vi "Modbus Master example merged.vi"() -> ()   [LabVIEW 2020, in "Modbus.lvlib"]
uses:
  Modbus.lvlib
  <vilib>/NI/Modbus Library/API/Master/Modbus Master.lvclass
  <vilib>/NI/Modbus Library/Master Function Definition/Read Device ID code.ctl
  <vilib>/NI/Modbus Library/API/Wrapper/Create TCP Master.vi
  <vilib>/NI/Modbus Library/API/Wrapper/API Main.lvlib
  <vilib>/NI/Modbus Library/Data Model/Device Data Model.lvclass
panel:
  out "Command PLC to spill gasoline can":bool
  out "Connected state":bool
  in  "Command PLC to spil gasoline can":bool
  in  "Holding Registers":u16[](array[numeric])=[0, 0, 0, 0, 0, 0, 0, 0]
  in  "Coils":bool[](array[boolean])=[FALSE, FALSE, FALSE, FALSE, FALSE, FALSE, FALSE, FALSE]
  out "Discrete Inputs":bool[](array[boolean])
  out "Input Registers":u16[](array[numeric])
  out "Basic Objects":string[](array[string])
  in  "Slave Address":string="localhost"
  in  "Port":u16=502
  out "Status":string
  in  "Stop Button":bool
  in  "Set Holding Registers":bool
  in  "Set Coils":bool
  in  "Fetch Discrete Inputs":bool
  in  "Fetch Input Registers":bool
  in  "Fetch Basic Objects":bool
  in  "Disconnect":bool
  in  "Connect":bool
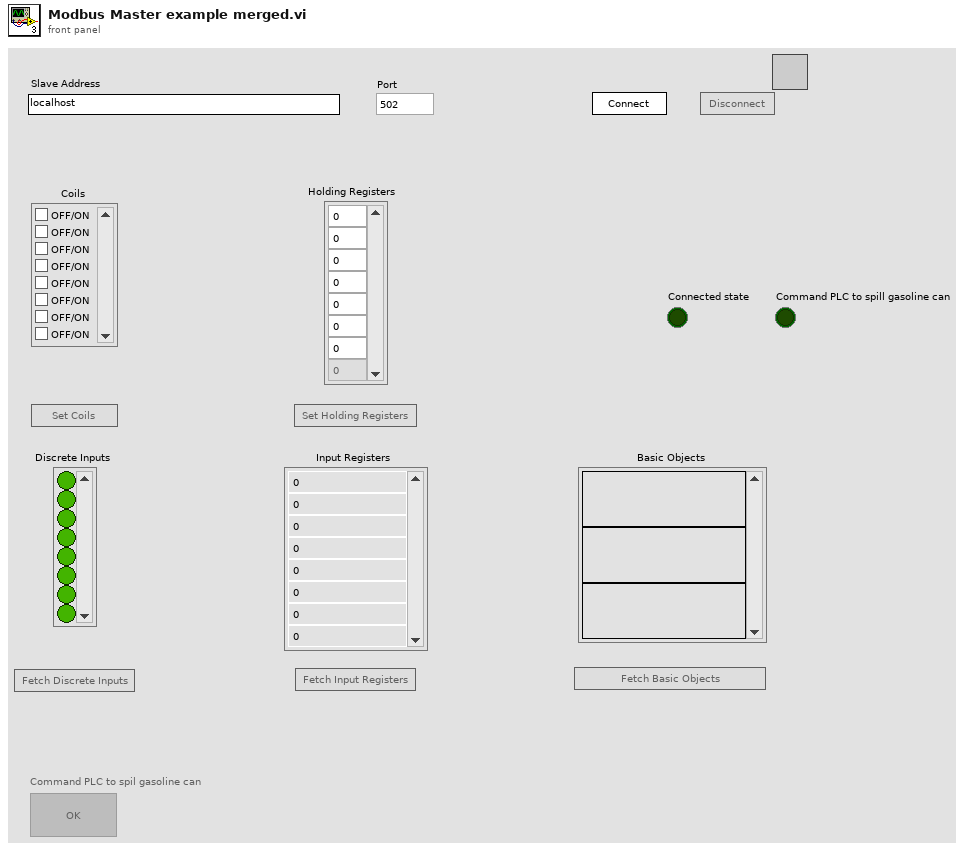
[diagram p1: front panel]
types:
  T1 = enum8{"Enabled", "Disabled", "Disabled and Grayed Out"}
  T2 = typedef "Device Data Model.lvclass/Read Device ID code.ctl" = enum8{"Read Basic", "Read Regular", "Read Extended", "Read Specific"}
  T3 = typedef "Device Data Model.lvclass/Identification Parameters.ctl" = cluster{"Object ID":u8, "Value":string}
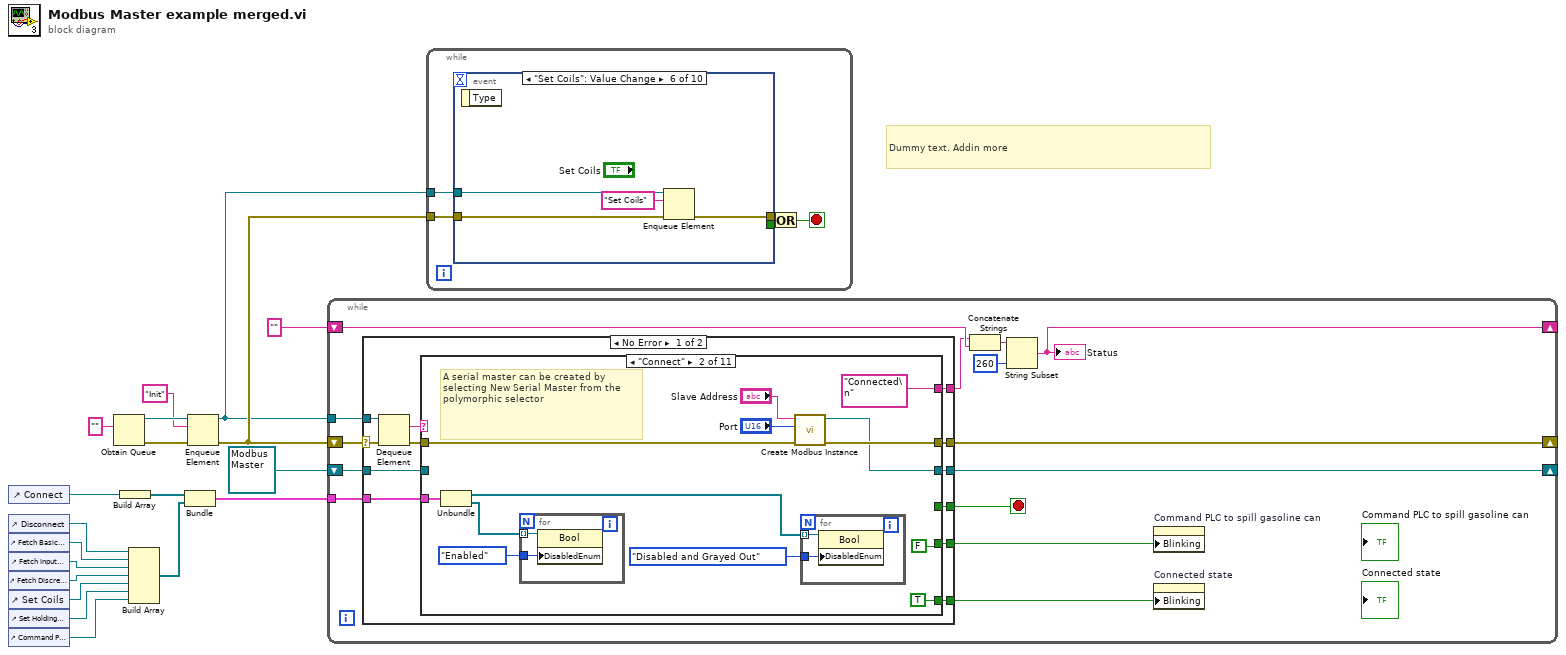
[diagram p0: block diagram]
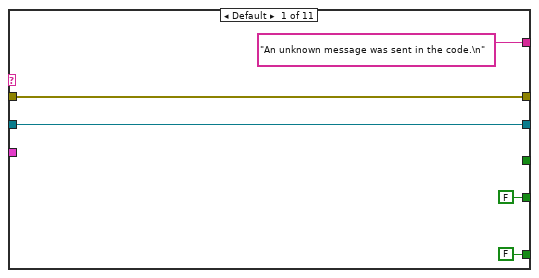
[diagram p2: hidden frame]
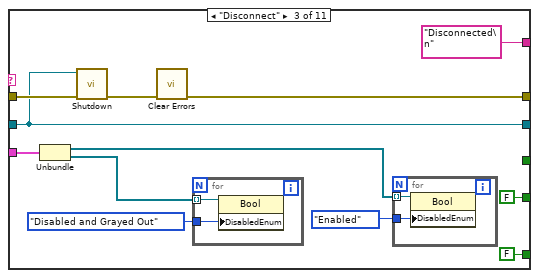
[diagram p3: hidden frame]
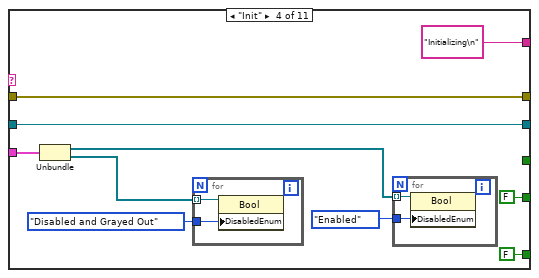
[diagram p4: hidden frame]
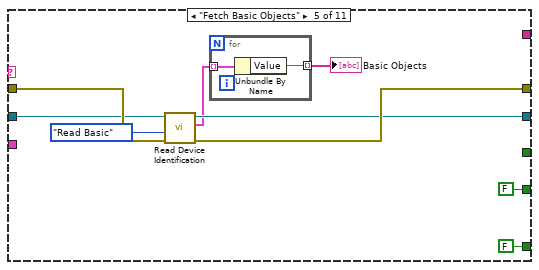
[diagram p5: hidden frame]
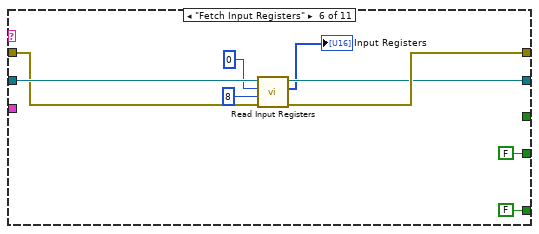
[diagram p6: hidden frame]
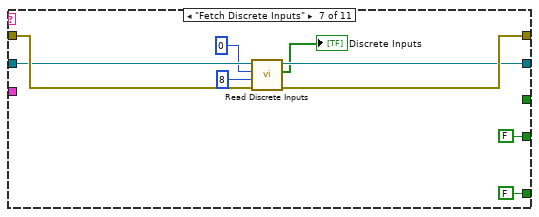
[diagram p7: hidden frame]
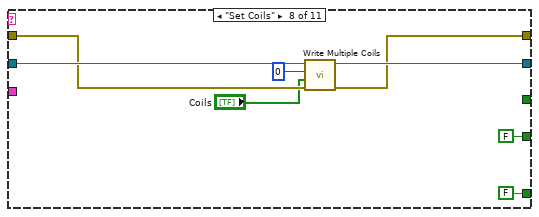
[diagram p8: hidden frame]
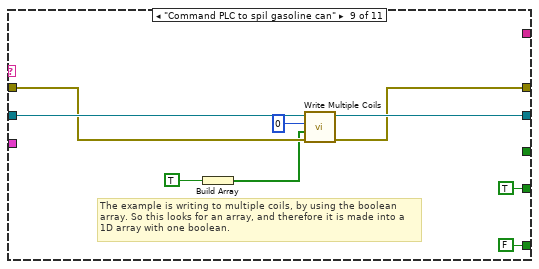
[diagram p9: hidden frame]
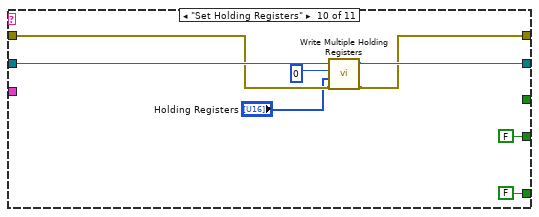
[diagram p10: hidden frame]
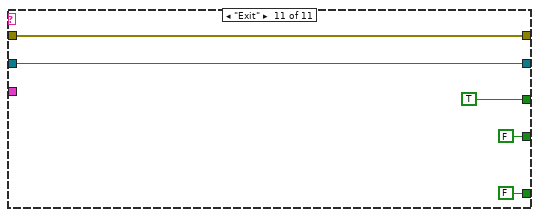
[diagram p11: hidden frame]
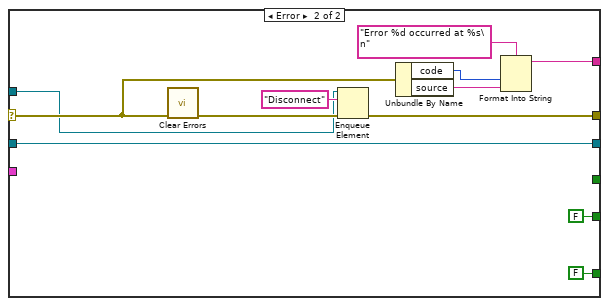
[diagram p12: hidden frame]
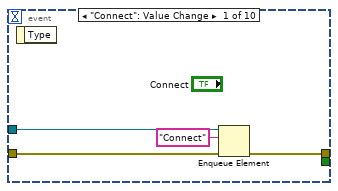
[diagram p13: hidden frame]
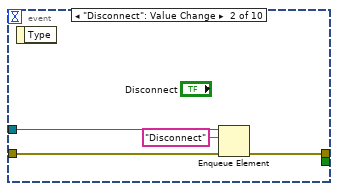
[diagram p14: hidden frame]
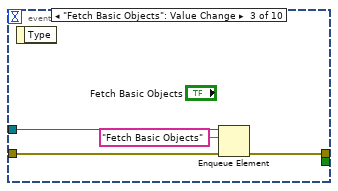
[diagram p15: hidden frame]
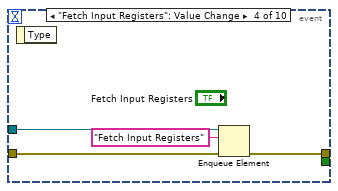
[diagram p16: hidden frame]
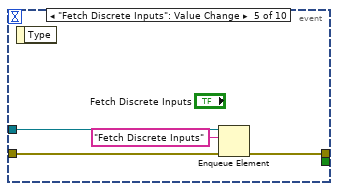
[diagram p17: hidden frame]
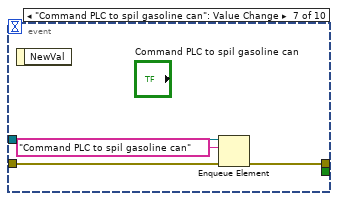
[diagram p18: hidden frame]
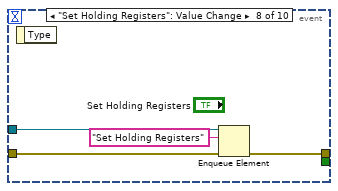
[diagram p19: hidden frame]
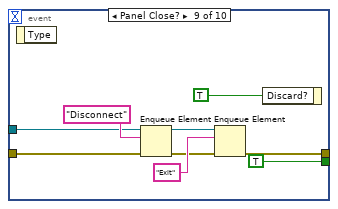
[diagram p20: hidden frame]
diagram:
  # "Dummy text. Addin more"
  n1 = control-ref of="Connect"() -> (w10:refnum<vi>)
  n2 = control-ref of="Disconnect"() -> (w16:refnum<vi>)
  n3 = control-ref of="Fetch Basic Objects"() -> (w15:refnum<vi>)
  n4 = control-ref of="Fetch Input Registers"() -> (w14:refnum<vi>)
  n5 = control-ref of="Fetch Discrete Inputs"() -> (w13:refnum<vi>)
  n6 = control-ref of="Set Coils"() -> (w12:refnum<vi>)
  n7 = control-ref of="Set Holding Registers"() -> (w11:refnum<vi>)
  n8 = control-ref of="Command PLC to spil gasoline can"() -> (w1:refnum<vi>)
  n9 = Obtain Queue(element data type="") -> (queue out=w5:refnum<queue>, error out=w19:errorcluster)  [unwired: 4 in, 1 out]
  n10 = Build Array(w10) -> (w7:refnum<vi>[])
  n11 = Build Array(w16, w15, w14, w13, w12, w11, w1) -> (w9:refnum<vi>[])
  n12 = Bundle(w7, w9) -> (w8:cluster{refnum<vi>[], refnum<vi>[]})  [unwired: 1 in]
  n13 = Enqueue Element(queue=w5, element="Init", error in (no error)=w19) -> (queue out=w4:refnum<queue>, error out=w6:errorcluster)  [unwired: 1 in, 1 out]
  n14 = while {
    shift-right: [w25] -> _
    shift-left: refnum<class "Modbus Master.lvclass"> refnum ("Modbus Master") -> [w24]
    tunnel: w4 -> [w33]
    shift-right: [w31] -> _
    shift-left: w6 -> [w32]
    shift-right: [w30] -> _
    shift-left: "" ("Status") -> [w27]
    tunnel: w8 -> [w22]
    stop <- w23 stop-if-true
    n15 = case shown="No Error" w32 {
      selector: w32 -> [w44 w166]
      tunnel: w33 -> [w45 w160]
      tunnel: [w41 w167] -> w31
      tunnel: [w38 w163] -> w26
      tunnel: [w40 w159] -> w25
      tunnel: w24 -> [w39 w159]
      tunnel: [w37 _] -> w23
      tunnel: w22 -> [w36 _]
      tunnel: [w35 FALSE] -> w21
      tunnel: [w34 FALSE ("Blinking")] -> w20
      frame No Error {
        n16 = Dequeue Element(queue=w45, error in (no error)=w44) -> (element=w42:string, error out=w43:errorcluster)  [unwired: 1 in, 2 out]
        n17 = case shown="\"Connect\"" w42 {
          tunnel: w43 -> [w50 w62 w79 w93 w106 w114 w126 w131 w140 w148 w156]
          tunnel: [w50 w61 w75 w93 w105 w117 w125 w132 w141 w149 w156] -> w41
          tunnel: [w49 w60 w77 w92 w103 w116 w123 w133 w142 w150 w155] -> w40
          tunnel: w39 -> [w49 _ w77 w92 w104 w115 w124 w134 w143 w151 w155]
          tunnel: ["An unknown message was sent in the code.\n" "Connected\n" "Disconnected\n" "Initializing\n" _ _ _ _ _ _ _] -> w38
          tunnel: [_ _ _ _ _ _ _ _ _ _ TRUE] -> w37
          tunnel: w36 -> [_ w58 w74 w90 _ _ _ _ _ _ _]
          tunnel: [FALSE TRUE FALSE FALSE FALSE FALSE FALSE FALSE FALSE FALSE FALSE] -> w35
          tunnel: [FALSE ("Blinking") FALSE ("Blinking") FALSE ("Blinking") FALSE ("Blinking") FALSE ("Blinking") FALSE ("Blinking") FALSE ("Blinking") FALSE ("Blinking") TRUE ("Blinking") FALSE ("Blinking") FALSE ("Blinking")] -> w34
          frame Default {
          }
          frame "Connect" {
            # "A serial master can be created by selecting New Serial Master from the polymorphic selector"
            n18 = Unbundle(w58) -> (w56:refnum<vi>[], w57:refnum<vi>[])
            n19 = for {
              tunnel: w57 -> [w65] mode=indexing
              tunnel: T1."Enabled" ("Disabled") -> [w64]
              n20 = property class="Bool"(reference=w65, "DisabledEnum"=w64) -> ()  [unwired: 1 in, 2 out]
            }
            n21 = call-poly <vilib>:"Create Modbus Instance.vi"("error in"=w62, "port (502)"="Port", "address"="Slave Address") -> ("error out"=w61:errorcluster, "TCP master instance"=w60:refnum<class "Modbus Master.lvclass">)  [unwired: 7 in]
            n22 = for {
              tunnel: w56 -> [w67] mode=indexing
              tunnel: T1."Disabled and Grayed Out" ("Disabled") -> [w66]
              n23 = property class="Bool"(reference=w67, "DisabledEnum"=w66) -> ()  [unwired: 1 in, 2 out]
            }
          }
          frame "Disconnect" {
            n24 = Unbundle(w74) -> (w72:refnum<vi>[], w73:refnum<vi>[])
            n25 = call-dynamic "Shutdown.vi"("error in"=w79, "Modbus master in"=w77) -> ("error out"=w78:errorcluster)  [unwired: 9 in]
            n26 = call <vilib>:"Clear Errors.vi"("error in (no error)"=w78) -> ("error out"=w75:errorcluster)  [unwired: 5 in, 1 out]
            n27 = for {
              tunnel: w73 -> [w83] mode=indexing
              tunnel: T1."Disabled and Grayed Out" ("Disabled") -> [w82]
              n28 = property class="Bool"(reference=w83, "DisabledEnum"=w82) -> ()  [unwired: 1 in, 2 out]
            }
            n29 = for {
              tunnel: w72 -> [w81] mode=indexing
              tunnel: T1."Enabled" ("Disabled") -> [w80]
              n30 = property class="Bool"(reference=w81, "DisabledEnum"=w80) -> ()  [unwired: 1 in, 2 out]
            }
          }
          frame "Init" {
            n31 = Unbundle(w90) -> (w88:refnum<vi>[], w89:refnum<vi>[])
            n32 = for {
              tunnel: w89 -> [w97] mode=indexing
              tunnel: T1."Disabled and Grayed Out" ("Disabled") -> [w96]
              n33 = property class="Bool"(reference=w97, "DisabledEnum"=w96) -> ()  [unwired: 1 in, 2 out]
            }
            n34 = for {
              tunnel: w88 -> [w95] mode=indexing
              tunnel: T1."Enabled" ("Disabled") -> [w94]
              n35 = property class="Bool"(reference=w95, "DisabledEnum"=w94) -> ()  [unwired: 1 in, 2 out]
            }
          }
          frame "Fetch Basic Objects" {
            n36 = call-dynamic "Read Device Identification.vi"("error in"=w106, "read device ID code"=Read_Device_ID_code."Read Basic" ("Read Device ID code"), "Modbus master in"=w104) -> ("error out"=w105:errorcluster, "objects"=w101:T3[], "Modbus master out"=w103:refnum<class "Modbus Master.lvclass">)  [unwired: 6 in]
            n37 = for {
              tunnel: w101 -> [w108] mode=indexing
              tunnel: [w107] -> w100 mode=indexing
              n38 = Unbundle By Name(w108) -> ("Value"=w107:string)
            }
            "Basic Objects" <- w100
          }
          frame "Fetch Input Registers" {
            n39 = call-dynamic "Read Input Registers.vi"("error in"=w114, "number of inputs"=u16 8 ("number of registers"), "starting address"=u16 0, "Modbus master in"=w115) -> ("error out"=w117:errorcluster, "register values"=→"Input Registers":u16[], "Modbus master out"=w116:refnum<class "Modbus Master.lvclass">)  [unwired: 5 in]
          }
          frame "Fetch Discrete Inputs" {
            n40 = call-dynamic "Read Discrete Inputs.vi"("error in"=w126, "number of inputs"=u16 8, "starting address"=u16 0, "Modbus master in"=w124) -> ("error out"=w125:errorcluster, "discrete inputs"=→"Discrete Inputs":bool[], "Modbus master out"=w123:refnum<class "Modbus Master.lvclass">)  [unwired: 5 in]
          }
          frame "Set Coils" {
            n41 = call-dynamic "Write Multiple Coils.vi"("error in"=w131, "coils to write"="Coils", "starting address"=u16 0, "Modbus master in"=w134) -> ("error out"=w132:errorcluster, "Modbus master out"=w133:refnum<class "Modbus Master.lvclass">)  [unwired: 6 in]
          }
          frame "Command PLC to spil gasoline can" {
            # "The example is writing to multiple coils, by using the boolean array. So this looks for an array, and therefore it is made into a 1D array with one boolean."
            n42 = Build Array(TRUE) -> (w137:bool[])
            n43 = call-dynamic "Write Multiple Coils.vi"("error in"=w140, "coils to write"=w137, "starting address"=u16 0, "Modbus master in"=w143) -> ("error out"=w141:errorcluster, "Modbus master out"=w142:refnum<class "Modbus Master.lvclass">)  [unwired: 6 in]
          }
          frame "Set Holding Registers" {
            n44 = call-dynamic "Write Multiple Holding Registers.vi"("error in"=w148, "registers to write"="Holding Registers", "starting address"=u16 0, "Modbus master in"=w151) -> ("error out"=w149:errorcluster, "Modbus master out"=w150:refnum<class "Modbus Master.lvclass">)  [unwired: 6 in]
          }
          frame "Exit" {
          }
        }
      }
      frame Error {
        n45 = call <vilib>:"Clear Errors.vi"("error in (no error)"=w166) -> ("error out"=w168:errorcluster)  [unwired: 5 in, 1 out]
        n46 = Enqueue Element(queue=w160, element="Disconnect", error in (no error)=w168) -> (error out=w167:errorcluster)  [unwired: 1 in, 2 out]
        n47 = Unbundle By Name(w166) -> ("code"=w165:i32, "source"=w164:string)
        n48 = Format Into String(format string="Error %d occurred at %s\n", w165, w164) -> (resulting string=w163:string)  [unwired: 2 in, 1 out]
      }
    }
    n49 = Concatenate Strings(w26, w27) -> (w28:string)
    n50 = String Subset(string=w28, length (rest)=260 ("length (rest)")) -> (substring=w30:string)  [unwired: 1 in]
    "Status" <- w30
    n51 = property on="Command PLC to spill gasoline can" class="Bool (strict)"("Blinking"=w20) -> ()  [unwired: 2 in, 2 out]
    n52 = property on="Connected state" class="Bool (strict)"("Blinking"=w21) -> ()  [unwired: 2 in, 2 out]
  }
  n53 = while {
    tunnel: w6 -> [w173]
    tunnel: w4 -> [w172]
    stop <- w169 stop-if-true
    n54 = event shown="[5] \"Set Coils\": Value Change" {
      selector: _ -> [_ _ _ _ _ _ _ _ _ _]
      dyn-events: _ -> [_ _ _ _ _ _ _ _ _ _]
      timeout: _ -> [_ _ _ _ _ _ _ _ _ _]
      tunnel: w173 -> [w177 w181 w185 w189 w193 w197 w201 w205 w211 w220]
      tunnel: [w176 w180 w184 w188 w192 w196 w200 w204 w206 w215] -> w171
      tunnel: w172 -> [w175 w179 w183 w187 w191 w195 w199 w203 w208 w217]
      tunnel: [_ _ _ _ _ _ _ _ TRUE ("Discard?") TRUE ("Discard?")] -> w170
      event "Connect": Value Change {
        n55 = event-data() -> ()  [unwired: 1 in, 1 out]
        n56 = Enqueue Element(queue=w175, element="Connect", error in (no error)=w177) -> (error out=w176:errorcluster)  [unwired: 1 in, 2 out]
      }
      event "Disconnect": Value Change {
        n57 = event-data() -> ()  [unwired: 1 in, 1 out]
        n58 = Enqueue Element(queue=w179, element="Disconnect", error in (no error)=w181) -> (error out=w180:errorcluster)  [unwired: 1 in, 2 out]
      }
      event "Fetch Basic Objects": Value Change {
        n59 = event-data() -> ()  [unwired: 1 in, 1 out]
        n60 = Enqueue Element(queue=w183, element="Fetch Basic Objects", error in (no error)=w185) -> (error out=w184:errorcluster)  [unwired: 1 in, 2 out]
      }
      event "Fetch Input Registers": Value Change {
        n61 = event-data() -> ()  [unwired: 1 in, 1 out]
        n62 = Enqueue Element(queue=w187, element="Fetch Input Registers", error in (no error)=w189) -> (error out=w188:errorcluster)  [unwired: 1 in, 2 out]
      }
      event "Fetch Discrete Inputs": Value Change {
        n63 = event-data() -> ()  [unwired: 1 in, 1 out]
        n64 = Enqueue Element(queue=w191, element="Fetch Discrete Inputs", error in (no error)=w193) -> (error out=w192:errorcluster)  [unwired: 1 in, 2 out]
      }
      event "Set Coils": Value Change {
        n65 = event-data() -> ()  [unwired: 1 in, 1 out]
        n66 = Enqueue Element(queue=w195, element="Set Coils", error in (no error)=w197) -> (error out=w196:errorcluster)  [unwired: 1 in, 2 out]
      }
      event "Command PLC to spil gasoline can": Value Change {
        n67 = event-data() -> ()  [unwired: 1 in, 1 out]
        n68 = Enqueue Element(queue=w199, element="Command PLC to spil gasoline can", error in (no error)=w201) -> (error out=w200:errorcluster)  [unwired: 1 in, 2 out]
      }
      event "Set Holding Registers": Value Change {
        n69 = event-data() -> ()  [unwired: 1 in, 1 out]
        n70 = Enqueue Element(queue=w203, element="Set Holding Registers", error in (no error)=w205) -> (error out=w204:errorcluster)  [unwired: 1 in, 2 out]
      }
      event Panel Close? {
        n71 = event-data() -> ()  [unwired: 1 in, 1 out]
        n72 = Enqueue Element(queue=w208, element="Disconnect", error in (no error)=w211) -> (queue out=w209:refnum<queue>, error out=w207:errorcluster)  [unwired: 1 in, 1 out]
        n73 = Enqueue Element(queue=w209, element="Exit", error in (no error)=w207) -> (error out=w206:errorcluster)  [unwired: 1 in, 2 out]
        n74 = event-data("Discard?"=TRUE) -> ()  [unwired: 1 in, 1 out]
      }
      event "Stop Button": Value Change {
        n75 = event-data() -> ()  [unwired: 1 in, 1 out]
        n76 = Enqueue Element(queue=w217, element="Disconnect", error in (no error)=w220) -> (queue out=w218:refnum<queue>, error out=w216:errorcluster)  [unwired: 1 in, 1 out]
        n77 = Enqueue Element(queue=w218, element="Exit", error in (no error)=w216) -> (error out=w215:errorcluster)  [unwired: 1 in, 2 out]
      }
    }
    n78 = Or(x=w171, y=w170) -> (x .or. y?=w169:bool)
  }
